vi "ChangeDriveMode.vi"(8 "error in (no error)":errorcluster, 9 "Output":dbl, 10 "Control Mode":T8=enum."Unchanged / Invalid", 11 "RobotDriveRef":T1={"RobotDriveDevRef"={"DevStatus"={"status"=FALSE, "code"=0, "source"=""}, "Motors[]"=[], "Square Inputs"=FALSE, "Max Output"=1.0}, "Control Mode"=enum."Unchanged / Invalid", "Motor Settings"={"Wheel Radius"=0.0, "Encoder Ticks Per Rev"=0.0, "Gear Ratio"=0.0, "ClimbRev"=0.0}, "Default Control Mode"=enum."Unchanged / Invalid"}) -> (0 "error out":errorcluster, 3 "RobotDriveRef Out":T1={"RobotDriveDevRef"={"DevStatus"={"status"=FALSE, "code"=0, "source"=""}, "Motors[]"=[], "Square Inputs"=FALSE, "Max Output"=1.0}, "Control Mode"=enum."Unchanged / Invalid", "Motor Settings"={"Wheel Radius"=0.0, "Encoder Ticks Per Rev"=0.0, "Gear Ratio"=0.0, "ClimbRev"=0.0}, "Default Control Mode"=enum."Unchanged / Invalid"})   [LabVIEW 2015]
uses:
  <vilib>/Rock Robotics/WPI/CAN/TalonSRX/WPI_CANTalonSRX_APIControlMode.ctl
  RobotDrive Type Def.ctl
  <vilib>/Rock Robotics/WPI/MotorControl/WPI_MotorControlDeviceRef.ctl
  <vilib>/Rock Robotics/WPI/MotorControl/WPI_MotorControlType.ctl
  <vilib>/Rock Robotics/SystemInterfaces/DIO/FPGA_DIOPWMChannel.ctl
  <vilib>/Rock Robotics/WPI/PWM/WPI_PWMDeadband.ctl
  <vilib>/Rock Robotics/WPI/CAN/Jaguar/SubVIs/WPI_CANJaguar_ControlMode.ctl
  Drive Motor Settings.ctl
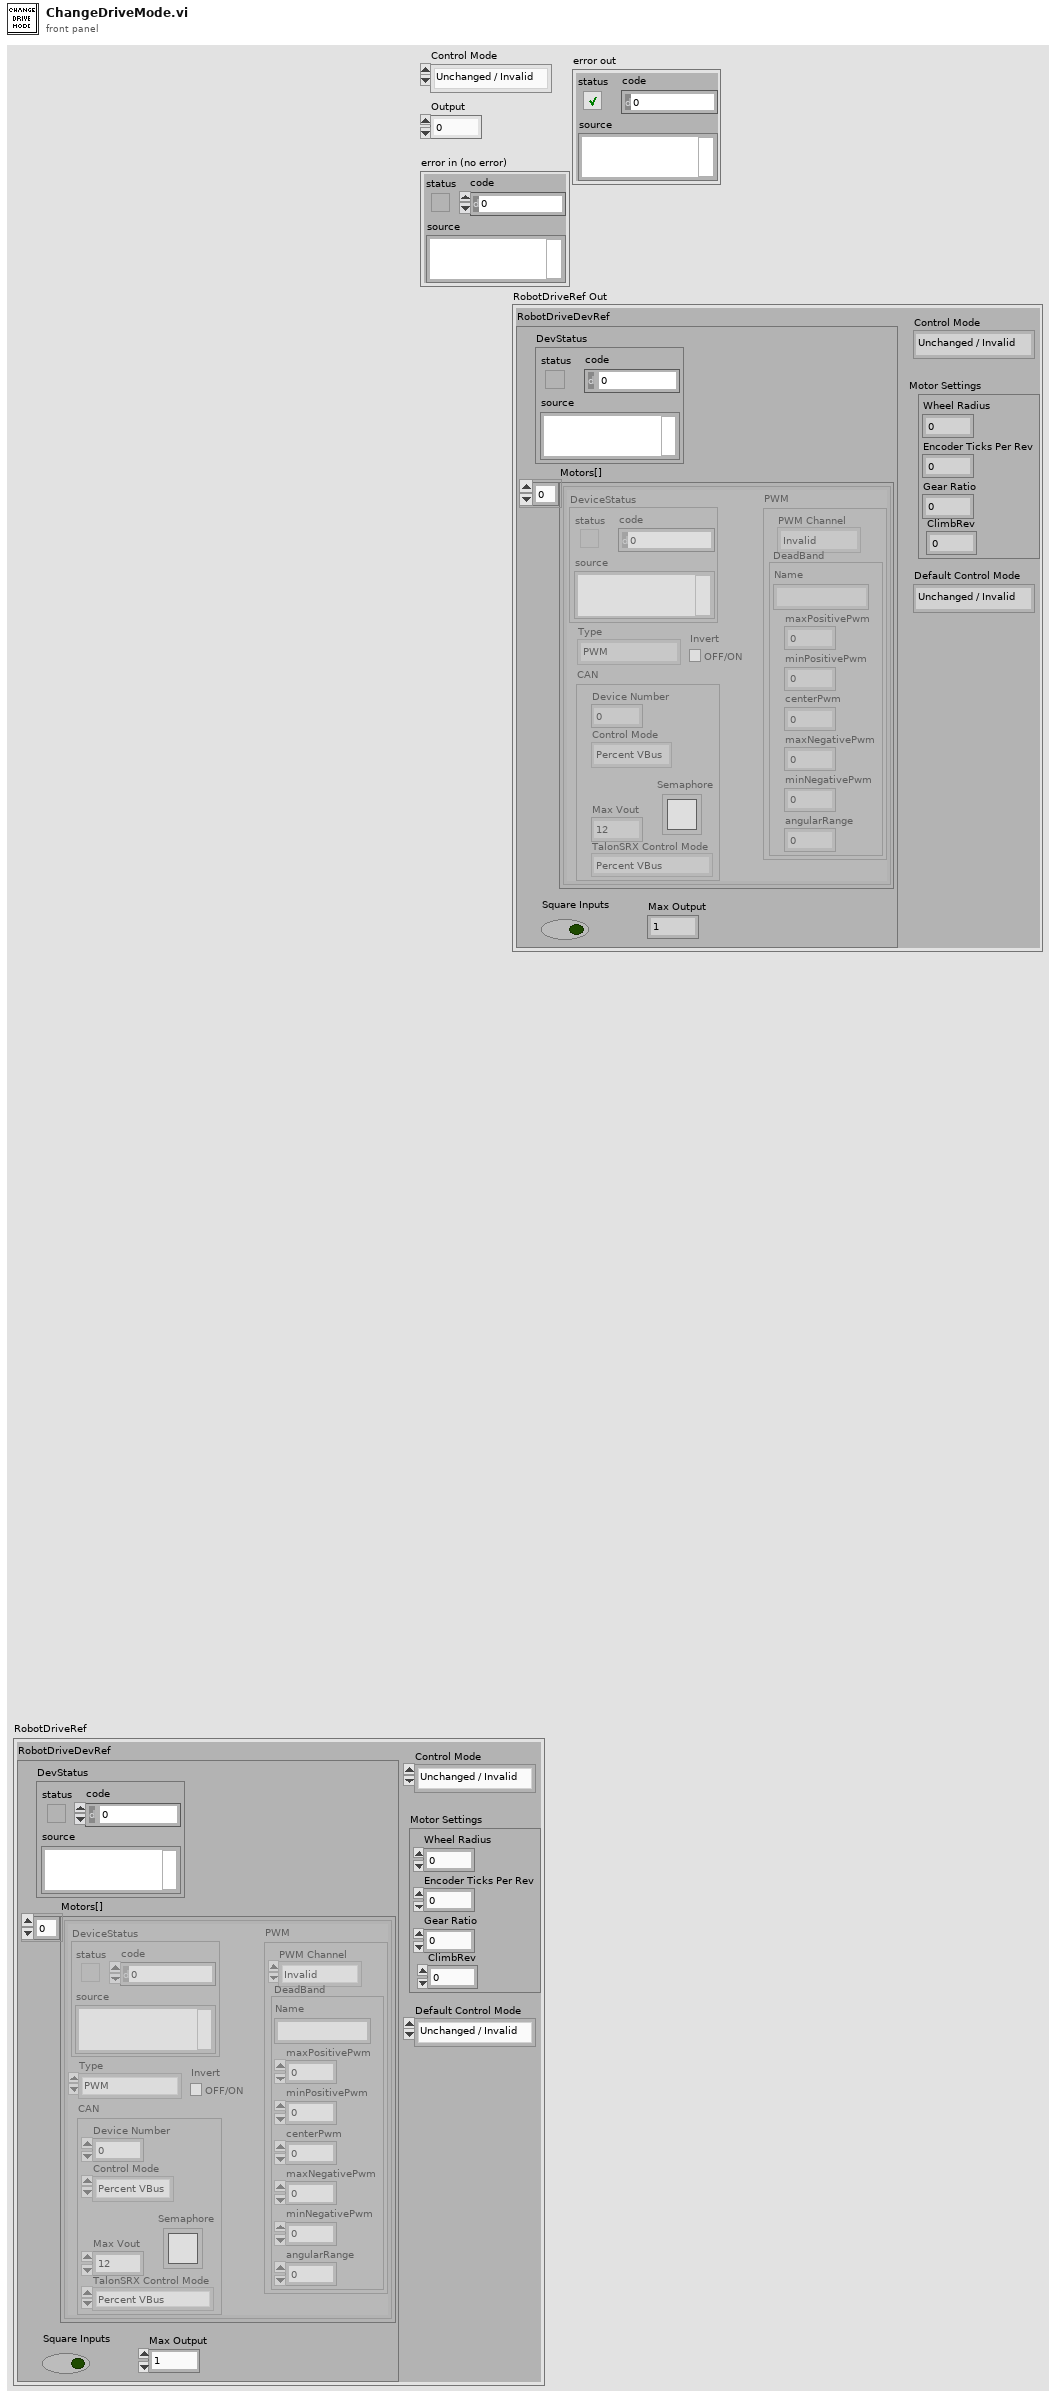
[diagram p1: front panel]
types:
  T1 = typedef "RobotDrive Type Def.ctl" = cluster{"RobotDriveDevRef":cluster{"DevStatus":errorcluster, "Motors[]":T2[], "Square Inputs":bool, "Max Output":dbl}, "Control Mode":T8, "Motor Settings":T9, "Default Control Mode":T8}
  T2 = typedef "WPI_MotorControlDeviceRef.ctl" = cluster{"DeviceStatus":errorcluster, "Type":T3, "PWM":cluster{"PWM Channel":T4, "DeadBand":T5}, "CAN":cluster{"Device Number":u8, "Control Mode":T6, "Semaphore":T7, "Max Vout":dbl, "TalonSRX Control Mode":T8}, "Invert":bool}
  T3 = typedef "WPI_MotorControlType.ctl" = enum16{"PWM", "CAN", "CANTalonSRX"}
  T4 = typedef "FPGA_DIOPWMChannel.ctl" = enum8{"PWM 0", "PWM 1", "PWM 2", "PWM 3", "PWM 4", "PWM 5", "PWM 6", "PWM 7", "PWM 8", "PWM 9", "PWM MXP 0", "PWM MXP 1", "PWM MXP 2", "PWM MXP 3", "PWM MXP 4", "PWM MXP 5", "PWM MXP 6", "PWM MXP 7", "PWM MXP 8", "PWM MXP 9", "Invalid"}
  T5 = typedef "WPI_PWMDeadband.ctl" = cluster{"Name":string, "maxPositivePwm":i32, "minPositivePwm":i32, "centerPwm":i32, "maxNegativePwm":i32, "minNegativePwm":i32, "angularRange":u16}
  T6 = typedef "WPI_CANJaguar_ControlMode.ctl" = enum8{"Percent VBus", "Current", "Speed", "Position", "Voltage"}
  T7 = typedef "Semaphore RefNum" = refnum<k1>
  T8 = typedef "WPI_CANTalonSRX_APIControlMode.ctl" = enum8{"Percent VBus", "Speed", "Position", "Slave", "Unchanged / Invalid", "Voltage Compensation", "Current", "Motion Profile"}
  T9 = typedef "Drive Motor Settings.ctl" = cluster{"Wheel Radius":dbl, "Encoder Ticks Per Rev":dbl, "Gear Ratio":dbl, "ClimbRev":dbl}
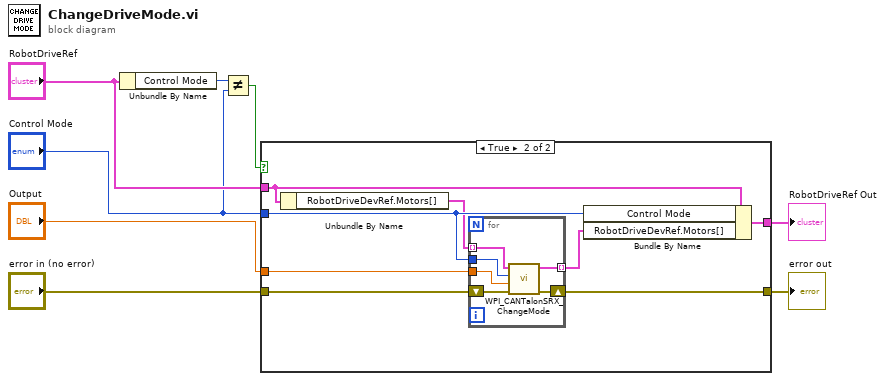
[diagram p0: block diagram]
diagram:
  n1 = Unbundle By Name("RobotDriveRef") -> ("Control Mode"=w3:T8)
  n2 = Not Equal?(x=w3, y="Control Mode") -> (x != y?=w1:bool)
  n3 = case shown="True" w1 {
    tunnel: "Output" -> [_ w18]
    tunnel: "error in (no error)" -> [w9 w17]
    tunnel: [w9 w16] -> w6
    tunnel: "Control Mode" -> [_ w15]
    tunnel: "RobotDriveRef" -> [w10 w12]
    tunnel: [w10 w14] -> w5
    frame False {
    }
    frame True {
      n4 = Unbundle By Name(w12) -> ("RobotDriveDevRef.Motors[]"=w11:T2[])
      n5 = for {
        tunnel: w11 -> [w20] mode=indexing
        tunnel: w15 -> [w24]
        tunnel: w18 -> [w23]
        shift-right: [w21] -> w16
        shift-left: w17 -> [w22]
        tunnel: [w19] -> w13 mode=indexing
        n6 = call <vilib>:"WPI_CANTalonSRX_ChangeMode.vi"("error in (no error)"=w22, "Output"=w23, "Control Mode"=w24, "CAN Talon SRX Ref"=w20) -> ("error out"=w21:errorcluster, "CAN Talon SRX Ref"=w19:T2)  [unwired: 6 in]
      }
      n7 = Bundle By Name(cluster=w12, "Control Mode"=w15, "RobotDriveDevRef.Motors[]"=w13) -> (w14:T1)
    }
  }
  "error out" <- w6
  "RobotDriveRef Out" <- w5
